vi "ENCODE.vi"(11 "Registers":u16[](array[numeric])) -> (3 "变体":variant)   [LabVIEW 2016, in "Primary Productivity.lvclass"]
uses:
  Primary Productivity.lvclass
panel:
  in  "错误输入":errorcluster
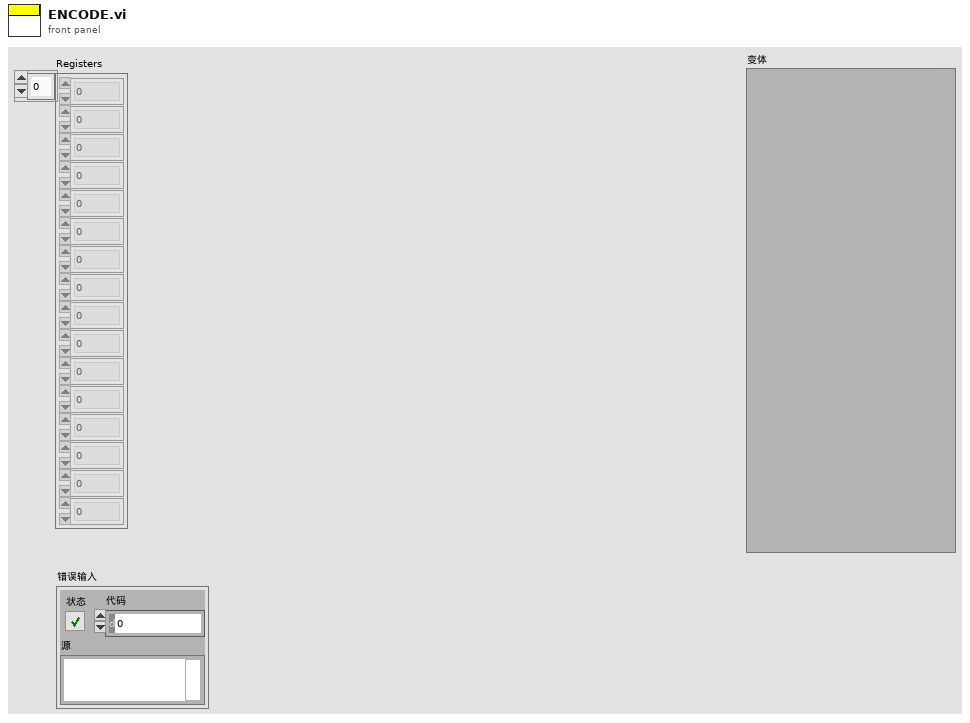
[diagram p1: front panel]
types:
  T1 = cluster{"name":string, "type":enum16{"int", "float", "string"}, "index":i32}[]
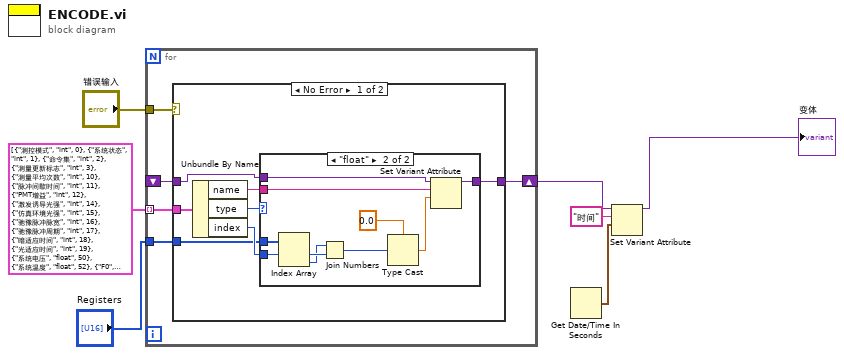
[diagram p0: block diagram]
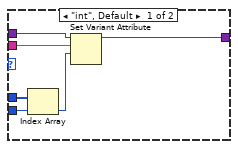
[diagram p2: hidden frame]
diagram:
  n1 = for {
    tunnel: T1 [{"name"="测控模式", "type"=enum."int", "index"=0}, {"name"="系统状态", "type"=enum."int", "index"=1}, {"name"="命令集", "type"=enum."int", "index"=2}, {"name"="测量更新标志", "type"=enum."int", "index"=3}, {"name"="测量平均次数", "type"=enum."int", "index"=10}, {"name"="脉冲间歇时间", "type"=enum."int", "index"=11}, {"name"="PMT增益", "type"=enum."int", "index"=12}, {"name"="激发诱导光强", "type"=enum."int", "index"=14}, {"name"="仿真环境光强", "type"=enum."int", "index"=15}, {"name"="驰豫脉冲脉宽", "type"=enum."int", "index"=16}, {"name"="驰豫脉冲周期", "type"=enum."int", "index"=17}, {"name"="暗适应时间", "type"=enum."int", "index"=18}, {"name"="光适应时间", "type"=enum."int", "index"=19}, {"name"="系统电压", "type"=enum."float", "index"=50}, {"name"="系统温度", "type"=enum."float", "index"=52}, {"name"="F0", "type"=enum."float", "index"=54}, {"name"="Fm", "type"=enum."float", "index"=56}, {"name"="Fv", "type"=enum."float", "index"=58}, {"name"="Fv/Fm", "type"=enum."float", "index"=60}, {"name"="σPSII", "type"=enum."float", "index"=62}, {"name"="τQA", "type"=enum."float", "index"=64}, {"name"="F0'", "type"=enum."float", "index"=66}, {"name"="Fm'", "type"=enum."float", "index"=68}, {"name"="Fv'", "type"=enum."float", "index"=70}, {"name"="Fv'/Fm'", "type"=enum."float", "index"=72}, {"name"="σPSII’", "type"=enum."float", "index"=74}, {"name"="τQA’", "type"=enum."float", "index"=76}, {"name"="Chla", "type"=enum."float", "index"=78}, {"name"="PAR", "type"=enum."float", "index"=80}, {"name"="GPP", "type"=enum."float", "index"=82}, {"name"="DF0", "type"=enum."float", "index"=84}, {"name"="DFv", "type"=enum."float", "index"=86}] -> [w12] mode=indexing
    shift-right: [w11] -> w4
    shift-left: _ -> [w10]
    tunnel: "Registers" -> [w9]
    tunnel: "错误输入" -> [w8]
    n2 = case shown="No Error" w8 {
      tunnel: w12 -> [w19 _]
      tunnel: [w16 w36] -> w11
      tunnel: w10 -> [w15 w36]
      tunnel: w9 -> [w13 _]
      frame No Error {
        n3 = Unbundle By Name(w19) -> ("name"=w17:string, "type"=w18:enum16{"int", "float", "string"}, "index"=w14:i32)
        n4 = case shown="\"float\"" w18 {
          tunnel: w17 -> [w25 w31]
          tunnel: [w24 w32] -> w16
          tunnel: w15 -> [w23 w33]
          tunnel: w13 -> [w22 w30]
          tunnel: w14 -> [w21 w29]
          frame "int", Default {
            n5 = Index Array(array=w22, index=w21) -> (element=w20:u16)
            n6 = Set Variant Attribute(Variant=w23, name=w25, value=w20) -> (Variant out=w24:variant)  [unwired: 1 in, 2 out]
          }
          frame "float" {
            n7 = Index Array(array=w30, index #1=w29) -> (element #1=w27:u16, element #2=w26:u16)  [unwired: 1 in]
            n8 = Join Numbers(hi=w26, lo=w27) -> ((hi.lo)=w35:u32)
            n9 = Type Cast(type=sgl 0.0, x=w35) -> (*(type *) &x=w28:sgl)
            n10 = Set Variant Attribute(Variant=w33, name=w31, value=w28) -> (Variant out=w32:variant)  [unwired: 1 in, 2 out]
          }
        }
      }
      frame Error {
      }
    }
  }
  n11 = Get Date/Time In Seconds() -> (seconds since 1Jan1904=w1:timestamp)
  n12 = Set Variant Attribute(Variant=w4, name="时间" ("名称"), value=w1) -> (Variant out=→"变体":variant)  [unwired: 1 in, 2 out]
